vi "linetools.vi"(0 "X1":i32, 5 "Y1":i32, 7 "X2":i32, 9 "Y2":i32, 11 "error in (no error)":errorcluster) -> (4 "output cluster":T1, 15 "error out":errorcluster)   [LabVIEW 2014]
panel:
  in  "ROI Descriptor":T1={"Global Rectangle"=[2, 196, 507, 199], "Contours"=[{"ID"=enum."External", "Type"=2, "Coordinates"=[2, 198, 506, 196]}]} {"Contours"."Type" items=["No Selection", "Point", "Line", "Rectangle", "Oval", "Polygon", "Freehand Region", "Annulus", "Unused2", "Unused3", "Broken Line", "Freehand Line", "Rotated Rectangle"]}
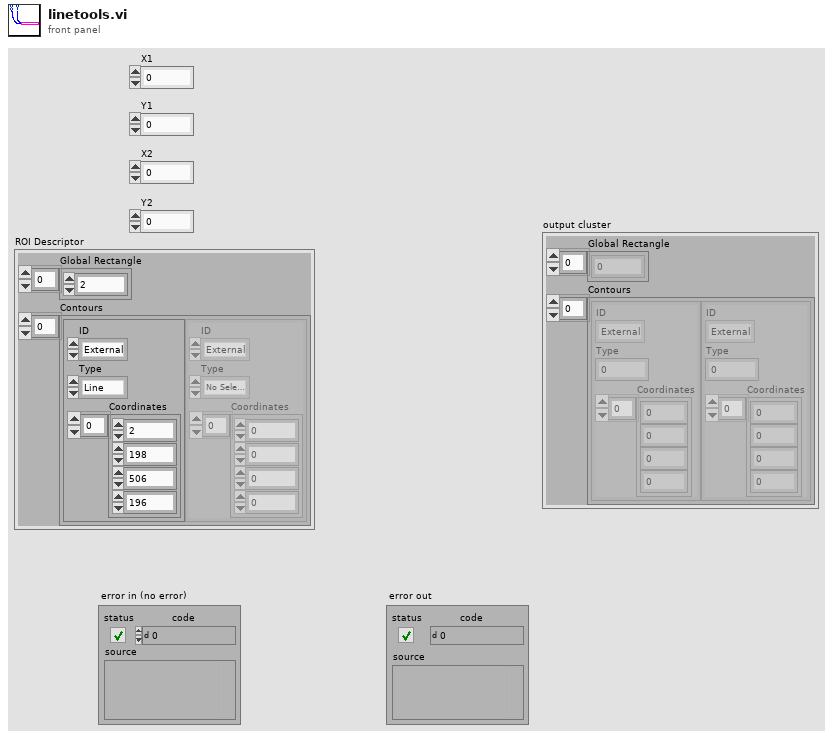
[diagram p1: front panel]
types:
  T1 = cluster{"Global Rectangle":i32[], "Contours":cluster{"ID":enum32{"External", "Internal"}, "Type":u32, "Coordinates":i32[]}[]}
  T2 = cluster{"ID":enum32{"External", "Internal"}, "Type":u32, "Coordinates":i32[]}[]
  T3 = cluster{"ID":enum32{"External", "Internal"}, "Type":u32, "Coordinates":i32[]}
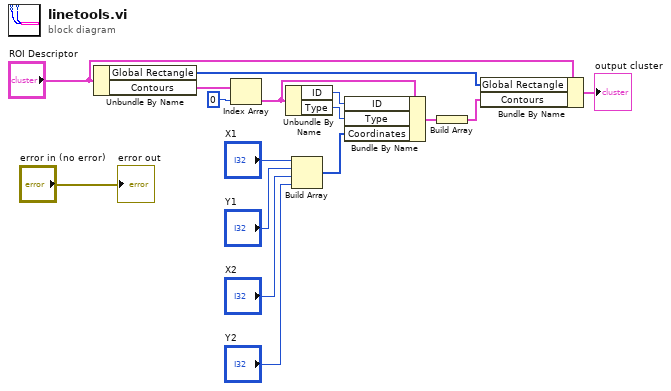
[diagram p0: block diagram]
diagram:
  n1 = Unbundle By Name("ROI Descriptor") -> ("Global Rectangle"=w3:i32[], "Contours"=w16:T2)
  n2 = Index Array(array=w16, index=0) -> (element=w7:T3)
  n3 = Unbundle By Name(w7) -> ("ID"=w14:enum32{"External", "Internal"}, "Type"=w13:u32)
  n4 = Build Array("X1", "Y1", "X2", "Y2") -> (w8:i32[])
  n5 = Bundle By Name(cluster=w7, "ID"=w14, "Type"=w13, "Coordinates"=w8) -> (w5:T3)
  n6 = Build Array(w5) -> (w4:T2)
  n7 = Bundle By Name(cluster="ROI Descriptor", "Global Rectangle"=w3, "Contours"=w4) -> (→"output cluster":T1)
  "error out" <- "error in (no error)"
